vi "Distribution_new.vi"(5 "Threshold":dbl, 6 "Baseline info 2":cluster{dbl[][]}[](array[cluster]), 7 "Event Detection (1D)":T1[](array[typedef])) -> (0 "Event final":dbl[][](array[numeric]), 2 "Baseline info OUT":cluster{dbl[][]}[](array[cluster]), 3 "Event Detection (1D) OUT":T1[](array[typedef]))   [LabVIEW 2017]
uses:
  <vilib>/Analysis/NI_AALPro.lvlib
  <vilib>/Analysis/NI_AALBase.lvlib
  Event Detection cluster.ctl
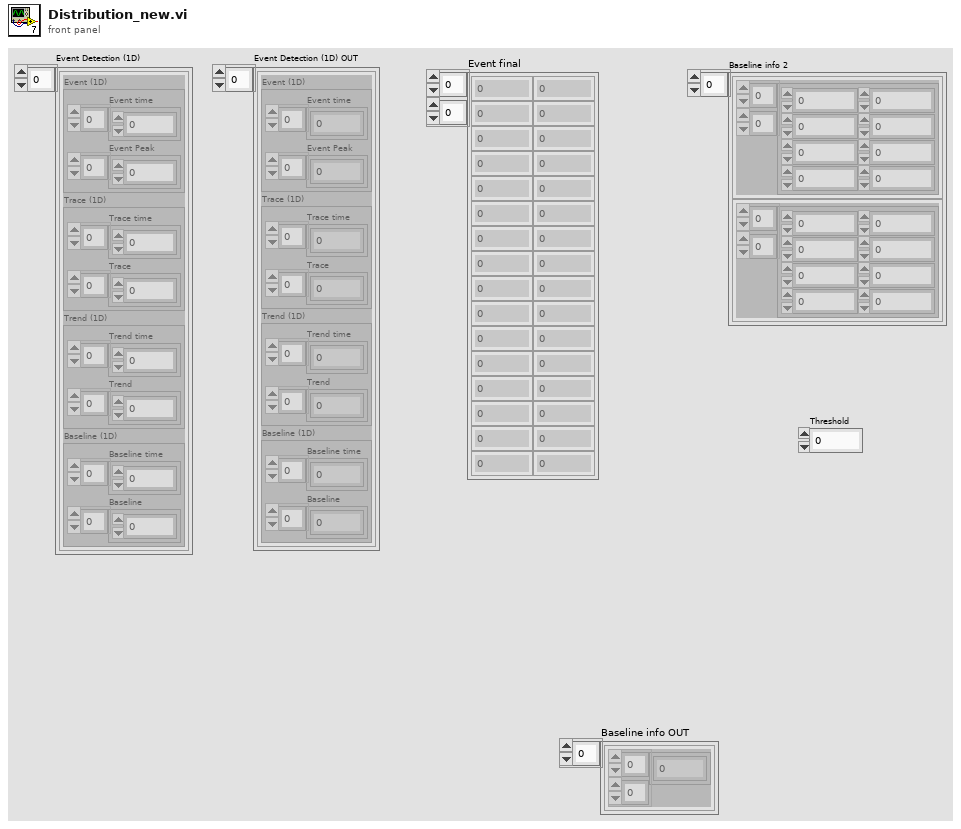
[diagram p1: front panel]
types:
  T1 = typedef "Event Detection cluster.ctl" = cluster{"Event (1D)":cluster{"Event time":dbl[], "Event Peak":dbl[]}, "Trace (1D)":cluster{"Trace time":dbl[], "Trace":dbl[]}, "Trend (1D)":cluster{"Trend time":dbl[], "Trend":dbl[]}, "Baseline (1D)":cluster{"Baseline time":dbl[], "Baseline":dbl[]}}
  T2 = cluster{"X Values":dbl[], "Histogram: h(x)":i32[]}
  T3 = cluster{string, "standard deviation":string, "standard deviation":string}
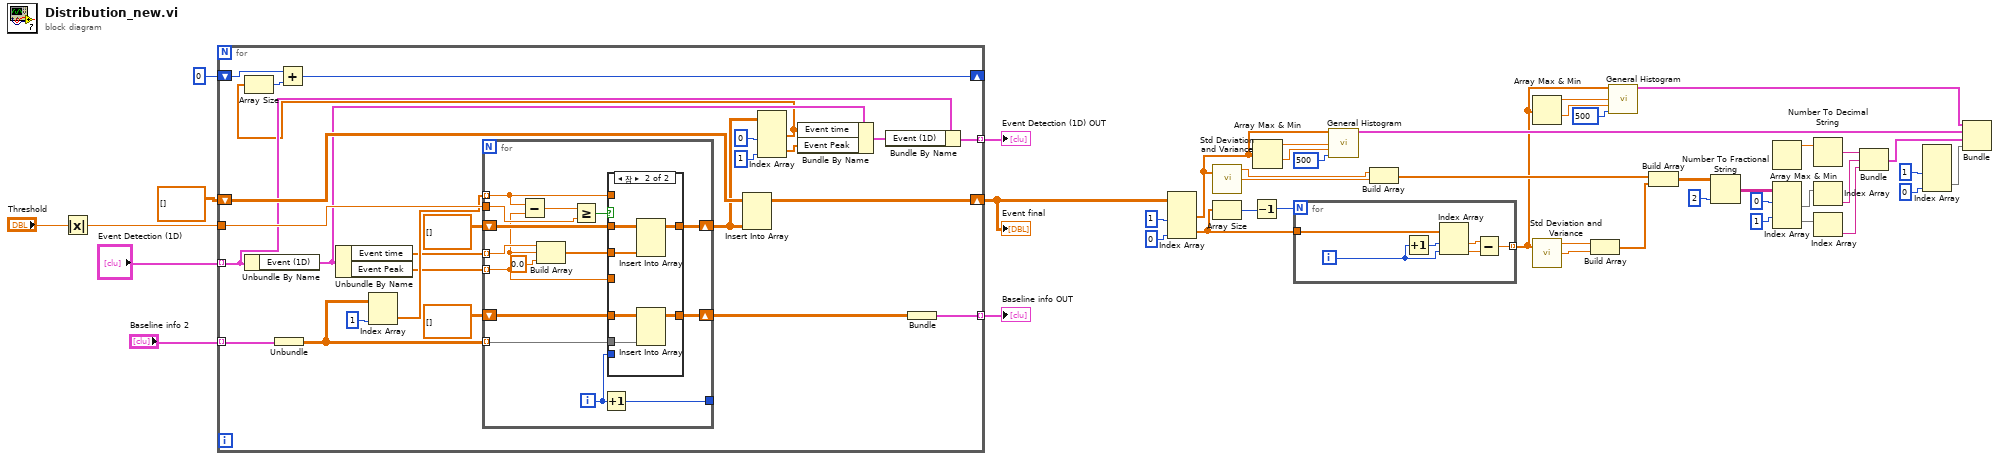
[diagram p0: block diagram]
diagram:
  n1 = Absolute Value(x="Threshold") -> (abs(x)=w10:dbl)
  n2 = for {
    tunnel: "Baseline info 2" -> [w70] mode=indexing
    shift-right: [w69] -> w38
    shift-left: dbl[][] [] -> [w68]
    shift-right: [w66] -> _
    shift-left: 0 ("인덱스") -> [w67]
    tunnel: w10 -> [w64]
    tunnel: [w61] -> w12 mode=indexing
    tunnel: "Event Detection (1D)" -> [w49] mode=indexing
    tunnel: [w47] -> w1 mode=indexing
    n3 = Unbundle By Name(w49) -> ("Event (1D)"=w52:cluster{"Event time":dbl[], "Event Peak":dbl[]})
    n4 = Unbundle(w70) -> (w50:dbl[][])
    n5 = Unbundle By Name(w52) -> ("Event time"=w57:dbl[], "Event Peak"=w56:dbl[])
    n6 = Index Array(array=w50, index (col)=1 ("비활성화된 인덱스 (열)")) -> (element=w58:dbl[])  [unwired: 1 in]
    n7 = for {
      tunnel: [w82] -> _
      tunnel: w58 -> [w72] mode=indexing
      shift-right: [w84] -> w55
      shift-left: dbl[][] [] -> [w83]
      tunnel: w64 -> [w80]
      shift-right: [w78] -> w62
      shift-left: dbl[][] [] -> [w77]
      tunnel: w57 -> [w74] mode=indexing
      tunnel: w56 -> [w73] mode=indexing
      tunnel: w50 -> [w71] mode=indexing
      i -> [w75]
      n8 = Subtract(x=w72, y=w73) -> (x-y=w81:dbl)
      n9 = Build Array(w74, w73, 0.0 ("원소")) -> (w85:dbl[])
      n10 = Greater Or Equal?(x=w81, y=w80) -> (x >= y?=w79:bool)
      n11 = Increment(x=w75) -> (x+1=w82:i32)
      n12 = case shown="참" w79 {
        tunnel: w85 -> [_ w93]
        tunnel: [w87 w92] -> w84
        tunnel: w83 -> [w87 w91]
        tunnel: [w86 w89] -> w78
        tunnel: w77 -> [w86 w90]
        tunnel: w75 -> [_ _]
        tunnel: w73 -> [_ _]
        tunnel: w72 -> [_ _]
        tunnel: w71 -> [_ w88]
        frame False {
        }
        frame True {
          n13 = Insert Into Array(array=w91, new element=w93) -> (w92:dbl[][])  [unwired: 2 in]
          n14 = Insert Into Array(array=w90, new element=w88) -> (w89:dbl[][])  [unwired: 2 in]
        }
      }
    }
    n15 = Insert Into Array(array=w68, new element=w55) -> (w69:dbl[][])  [unwired: 2 in]
    n16 = Index Array(array=w55, index (col) #1=0 ("비활성화된 인덱스 (열)"), index (col) #2=1 ("인덱스 (열)")) -> (element #1=w46:dbl[], element #2=w51:dbl[])  [unwired: 2 in]
    n17 = Array Size(array=w46) -> (size(s)=w60:i32)
    n18 = Add(x=w67, y=w60) -> (x+y=w66:i32)
    n19 = Bundle By Name(cluster=w52, "Event time"=w46, "Event Peak"=w51) -> (w48:cluster{"Event time":dbl[], "Event Peak":dbl[]})
    n20 = Bundle By Name(cluster=w49, "Event (1D)"=w48) -> (w47:T1)
    n21 = Bundle(w62) -> (w61:cluster{dbl[][]})  [unwired: 1 in]
  }
  "Event final" <- w38
  "Baseline info OUT" <- w12
  "Event Detection (1D) OUT" <- w1
  n22 = Index Array(array=w38, index (col) #1=1 ("비활성화된 인덱스 (열)"), index (col) #2=0 ("인덱스 (열)")) -> (element #1=w5:dbl[], element #2=w30:dbl[])  [unwired: 2 in]
  n23 = call <vilib>:"Std Deviation and Variance.vi"("X"=w5) -> ("mean"=w37:dbl, "standard deviation"=w36:dbl)  [unwired: 1 in, 1 out]
  n24 = Array Size(array=w30) -> (size(s)=w43:i32)
  n25 = Decrement(x=w43) -> (x-1=w42:i32)
  n26 = Array Max & Min(array=w5) -> (max value=w4:dbl, min value=w3:dbl)  [unwired: 2 out]
  n27 = for {
    N: w42 -> [_]
    tunnel: w30 -> [w99]
    tunnel: [w94] -> w8 mode=indexing
    i -> [w97]
    n28 = Increment(x=w97) -> (x+1=w98:i32)
    n29 = Index Array(array=w99, index #1=w98, index #2=w97) -> (element #1=w96:dbl, element #2=w95:dbl)
    n30 = Subtract(x=w96, y=w95) -> (x-y=w94:dbl)
  }
  n31 = call <vilib>:"General Histogram.vi"("X"=w5, "max"=w4, "min"=w3, "# bins"=500) -> ("Histogram Graph"=w15:T2)  [unwired: 7 in, 4 out]
  n32 = Build Array(w37, w36) -> (w32:dbl[])
  n33 = Array Max & Min(array=w8) -> (max value=w7:dbl, min value=w6:dbl)  [unwired: 2 out]
  n34 = call <vilib>:"Std Deviation and Variance.vi"("X"=w8) -> ("mean"=w34:dbl, "standard deviation"=w35:dbl)  [unwired: 1 in, 1 out]
  n35 = Build Array(w34, w35) -> (w33:dbl[])
  n36 = call <vilib>:"General Histogram.vi"("X"=w8, "max"=w7, "min"=w6, "# bins"=500) -> ("Histogram Graph"=w16:T2)  [unwired: 7 in, 4 out]
  n37 = Build Array(w32, w33) -> (w26:dbl[][])
  n38 = Number To Fractional String(number=w26, precision (6)=i16 2 ("폭(-)")) -> (F-format string=w24:string[][])  [unwired: 2 in]
  n39 = Array Max & Min() -> (max value=w27:dbl)  [unwired: 1 in, 3 out]
  n40 = Index Array(array=w24, index (row) #1=0 ("인덱스 (행)"), index (row) #2=1 ("인덱스 (행)")) -> (element #1=w21:string[], element #2=w20:string[])  [unwired: 2 in]
  n41 = Number To Decimal String(number=w27) -> (decimal integer string=w19:string)  [unwired: 1 in]
  n42 = Index Array(array=w21) -> (element=w18:string)  [unwired: 1 in]
  n43 = Index Array(array=w20) -> (element=w17:string)  [unwired: 1 in]
  n44 = Bundle(w19, "standard deviation"=w18, "standard deviation"=w17) -> (w14:T3)  [unwired: 1 in]
  n45 = Index Array(index (col) #1=1 ("비활성화된 인덱스 (열)"), index (col) #2=0 ("인덱스 (열)")) -> (element #2=w13)  [unwired: 3 in, 1 out]
  n46 = Bundle("Histogram Graph"=w16, "Histogram Graph"=w15, w14, w13) -> ()  [unwired: 1 in, 1 out]
